vi "NewController.vi"(6 "Database":refnum<class "Database.lvclass">, 8 "error in (no error)":errorcluster, 9 "Name('')":string, 10 "ID(\"\")":string, 11 "Admin_Actor in":refnum<class "Admin_Actor.lvclass">) -> (0 "error out":errorcluster, 3 "Admin_Actor out":refnum<class "Admin_Actor.lvclass">)   [LabVIEW 2015, in "Admin_Actor.lvlib" / "Admin_Actor.lvclass"]
uses:
  Admin_Actor.lvclass
  API/_Database/Database.lvclass
  Admin_Actor.lvclass/Admin_Actor.ctl
  Setting/g_setting.vi
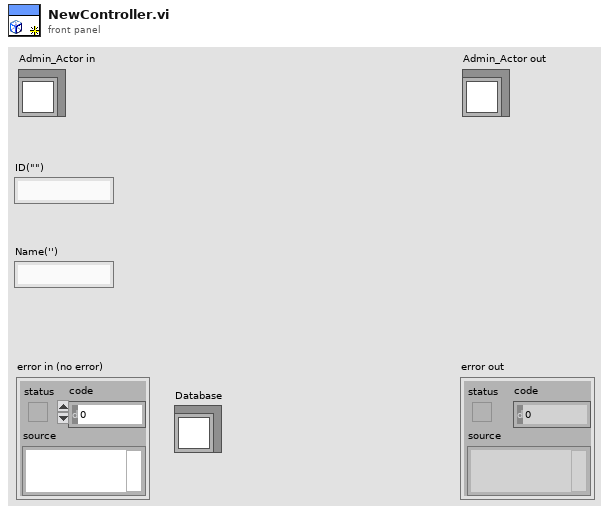
[diagram p1: front panel]
types:
  T1 = typedef "LVDateTimeRec.ctl" = cluster{"fractional second":dbl, "second":i32, "minute":i32, "hour":i32, "day of month":i32, "month":i32, "year":i32, "day of week":i32, "day of year":i32, "DST":i32}
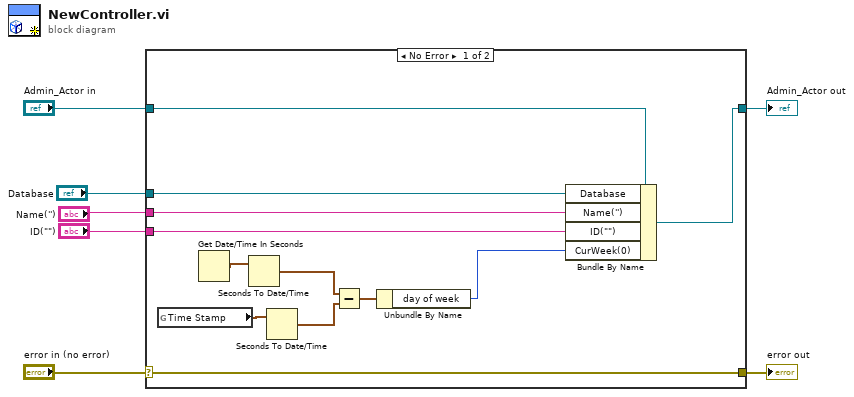
[diagram p0: block diagram]
diagram:
  n1 = case shown="No Error" "error in (no error)" {
    selector: "error in (no error)" -> [w19 w21]
    tunnel: [w19 w21] -> w6
    tunnel: [w17 w20] -> w4
    tunnel: "Admin_Actor in" -> [w18 w20]
    tunnel: "Database" -> [w16 _]
    tunnel: "Name('')" -> [w15 _]
    tunnel: "ID(\"\")" -> [w14 _]
    frame No Error {
      n2 = global read "g_setting.vi" "Time Stamp"() -> (w13:timestamp)
      n3 = Get Date/Time In Seconds() -> (seconds since 1Jan1904=w9:timestamp)
      n4 = Seconds To Date/Time(time stamp (now)=w9) -> (date time rec=w12:T1)  [unwired: 1 in]
      n5 = Seconds To Date/Time(time stamp (now)=w13) -> (date time rec=w11:T1)  [unwired: 1 in]
      n6 = Subtract(x=w12, y=w11) -> (x-y=w10:T1)
      n7 = Unbundle By Name(w10) -> ("day of week"=w8:i32)
      n8 = Bundle By Name(cluster=w18, "Database"=w16, "Name('')"=w15, "ID(\"\")"=w14, "CurWeek(0)"=w8) -> (w17:refnum<class "Admin_Actor.lvclass">)
    }
    frame Error {
    }
  }
  "error out" <- w6
  "Admin_Actor out" <- w4
